vi "Send Window Direct Message.vi"(7 "Message Priority (Normal)":T2=enum."Normal", 8 "error in (no error)":errorcluster, 10 "Message Cluster":T1, 11 "Message Enqueuer":refnum<class "Message Enqueuer.lvclass">) -> (0 "error out":errorcluster, 3 "Message Enqueuer out":refnum<class "Message Enqueuer.lvclass">)   [LabVIEW 2020, in "Interface.lvlib" / "Window Direct Message Msg.lvclass"]
doc: "This VI sends the message to an actor."
uses:
  Window Direct Message Msg.lvclass
  <vilib>/ActorFramework/Message Enqueuer/Message Enqueuer.lvclass
  <vilib>/ActorFramework/Message Enqueuer/Message Priority.ctl
  Application Control/Message.ctl
  C:/Program Files (x86)/National Instruments/LabVIEW 2020/vi.lib/ActorFramework/Message/Message.lvclass
  Window Direct Message Msg.lvclass/Window Direct Message Msg.ctl
  <vilib>/ActorFramework/Message Enqueuer/Message Enqueuer.lvclass/Message Enqueuer.ctl
  <vilib>/ActorFramework/Message Priority Queue/Priority Enqueue.vi
  F:/Gitlab Repository/LabVIEW-Study/10.Top 5 Actor Framework Overrides/Chat Room with Interface/Interface/Chat Room Window Messages/Window Direct Message Msg/Window Direct Message Msg.lvclass
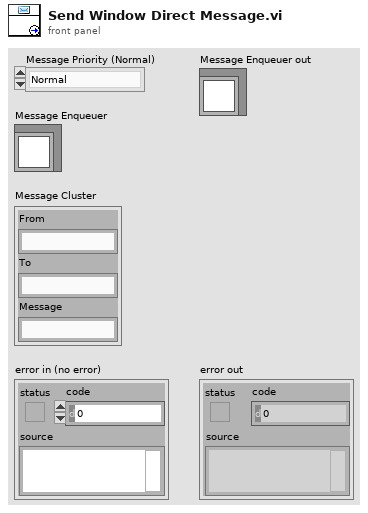
[diagram p1: front panel]
types:
  T1 = typedef "Message.ctl" = cluster{"From":string, "To":string, "Message":string}
  T2 = typedef "Actor Framework.lvlib/Message Enqueuer.lvclass/Message Priority.ctl" = enum16{"Low", "Normal", "High"}
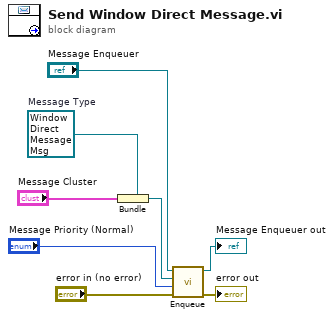
[diagram p0: block diagram]
diagram:
  w5 = refnum<class "Window Direct Message Msg.lvclass"> refnum  # Message Type
  n1 = Bundle(cluster=w5, "Message Cluster") -> (w4:refnum<class "Window Direct Message Msg.lvclass">)
  n2 = call <vilib>:"Enqueue.vi"("error in (no error)"="error in (no error)", "Message Priority (Normal)"="Message Priority (Normal)", "Message"=w4, "Message Enqueuer in"="Message Enqueuer") -> ("error out"=→"error out":errorcluster, "Message Enqueuer in"=→"Message Enqueuer out":refnum<class "Message Enqueuer.lvclass">)  [unwired: 6 in]
